vi "Write Owning System.vi"(8 "error in (no error)":errorcluster, 10 "Owning System":T1, 11 "Generic Hardware in":refnum<class "Generic Hardware.lvclass">) -> (0 "error out":errorcluster, 3 "Generic Hardware out":refnum<class "Generic Hardware.lvclass">)   [LabVIEW 2017, in "Generic Hardware.lvclass"]
uses:
  Generic Hardware.lvclass
  Type Defs/Owning System.ctl
  Generic Hardware.lvclass/Generic Hardware.ctl
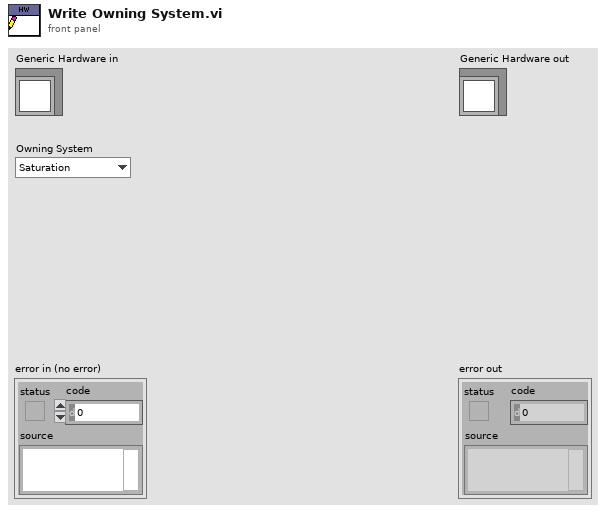
[diagram p1: front panel]
types:
  T1 = typedef "Generic Hardware.lvclass/Owning System.ctl" = enum16{"Saturation", "Expansion"}
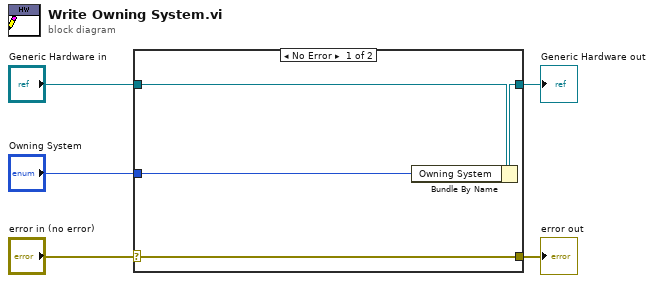
[diagram p0: block diagram]
diagram:
  n1 = case shown="No Error" "error in (no error)" {
    selector: "error in (no error)" -> [w9 w10]
    tunnel: [w9 w10] -> w4
    tunnel: [w7 w11] -> w2
    tunnel: "Generic Hardware in" -> [w8 w11]
    tunnel: "Owning System" -> [w6 _]
    frame No Error {
      n2 = Bundle By Name(cluster=w8, "Owning System"=w6) -> (w7:refnum<class "Generic Hardware.lvclass">)
    }
    frame Error {
    }
  }
  "error out" <- w4
  "Generic Hardware out" <- w2
